vi "Enable or Gray Control Refnum.vi"(8 "error in (no error)":errorcluster, 10 "enable?":bool, 11 "Control in":refnum<vi>) -> (0 "error out":errorcluster, 3 "Control out":refnum<vi>)   [LabVIEW 2020]
doc: "Uses a Boolean value to set a control refnum to \"Enabled\" (True) or to \"Disabed and Grayed\" (False)."
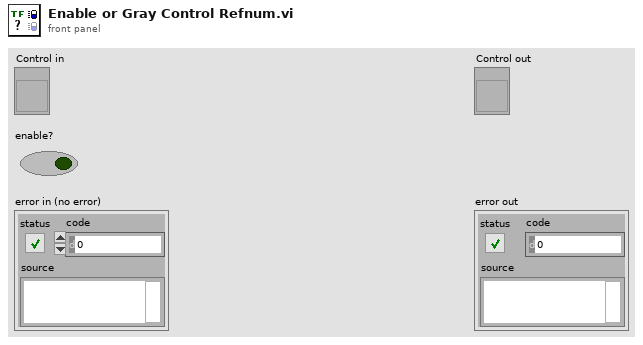
[diagram p1: front panel]
types:
  T1 = enum8{"Enabled", "Disabled", "Disabled and Grayed Out"}
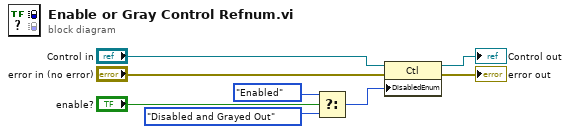
[diagram p0: block diagram]
diagram:
  n1 = Select(t=T1."Enabled" ("Disabled"), s="enable?", f=T1."Disabled and Grayed Out" ("Disabled")) -> (s? t:f=w5:T1)
  n2 = property on="Property Node" class="Ctl"(reference="Control in", error in="error in (no error)", "DisabledEnum"=w5) -> (reference out=→"Control out":refnum<vi>, error out=→"error out":errorcluster)
